vi "RT Main.vi"() -> ()   [LabVIEW 2014]
uses:
  controls/FPGA VI Reference.ctl
  Globals/Global - All RT Loop Stop.vi
  Globals/Global - Monitoring Variables.vi
  Globals/Global - Configuration Options.vi
  support/Message Queue/Message Queue.lvlib
  <vilib>/nisyscfg/nisyscfg.lvlib
  controls/Master Configuration.ctl
  controls/EPICS Configuration.ctl
panel:
  in  "Index":u32
  in  "Message":string
  in  "Send":bool
  in  "stop":bool
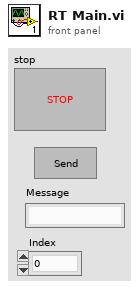
[diagram p1: front panel]
types:
  T1 = typedef "FPGA VI Reference.ctl" = refnum<k20>
  T2 = typedef "Master Configuration.ctl" = cluster{"Epics Configuration":T3, "Epics Configuration File":string, "Number of Channels":u8, "Data rate":u32, "PM Buffer Size":u32}
  T3 = typedef "EPICS Configuration.ctl" = cluster{"DIN Mask":bool[], "# Samples Post Trig":u32, "Armed":bool, "ADC Mask":bool[], "ADC Max Threshold":dbl[], "ADC Min Threshold":dbl[]}
  T4 = typedef "Message Queue.lvlib/All Real-Time Message Queues.ctl" = cluster{"Message Handler":refnum<queue>, "FPGA Subsystem":refnum<queue>}
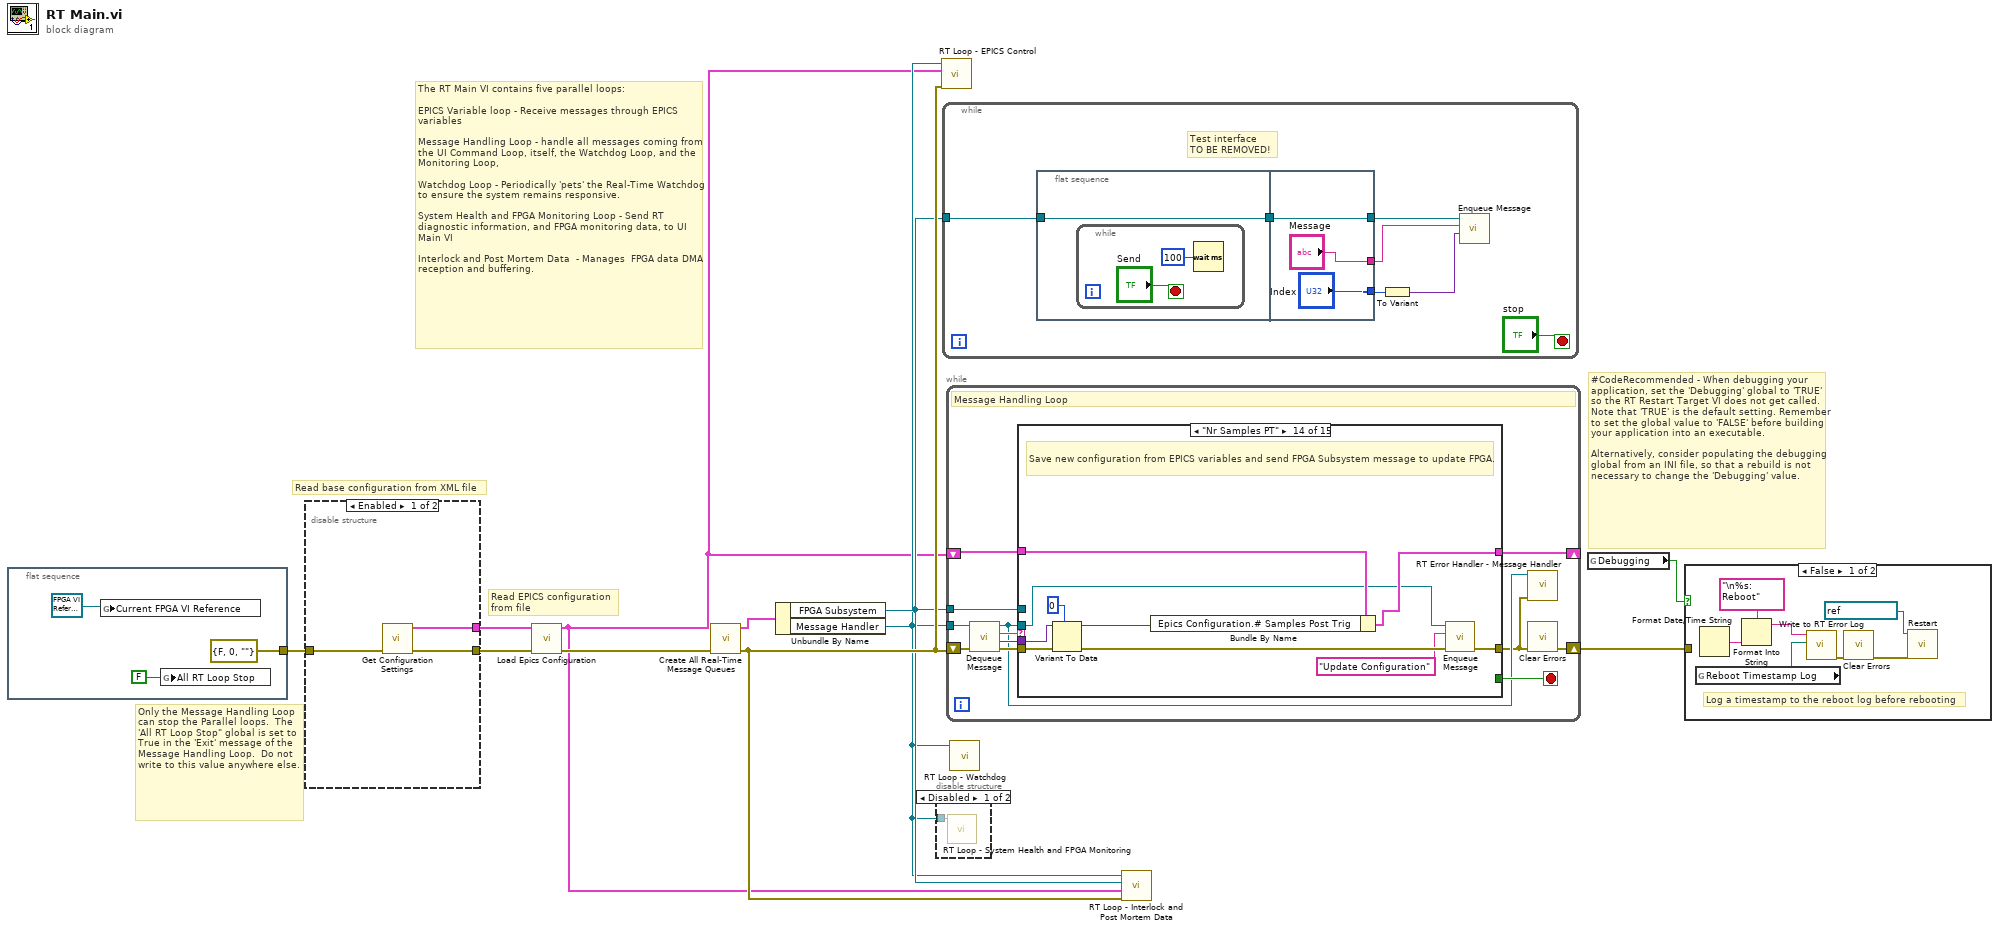
[diagram p0: block diagram]
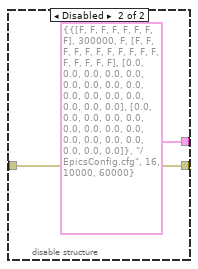
[diagram p3: hidden frame]
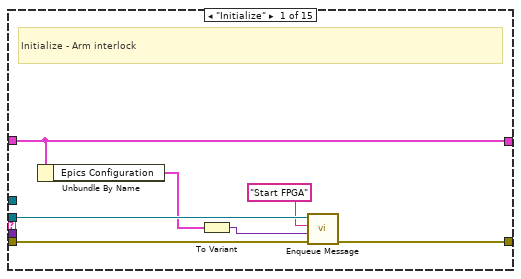
[diagram p5: hidden frame]
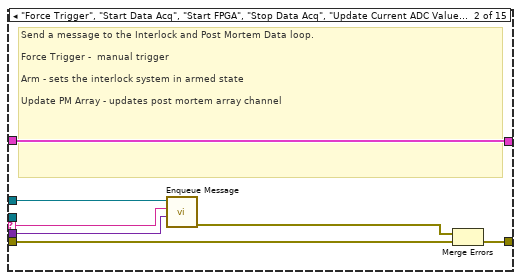
[diagram p6: hidden frame]
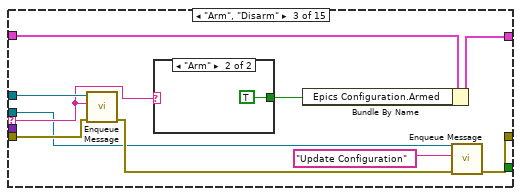
[diagram p7: hidden frame]
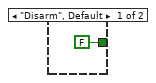
[diagram p8: hidden frame]
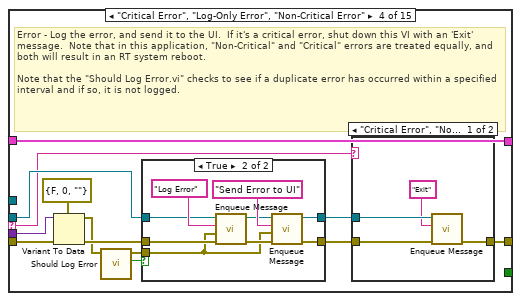
[diagram p9: hidden frame]
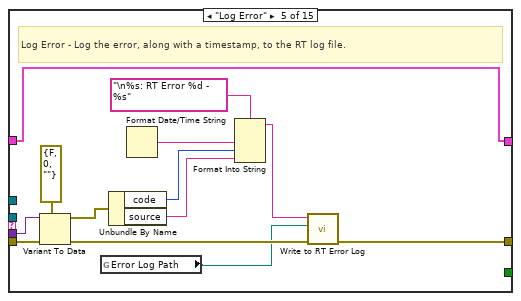
[diagram p12: hidden frame]
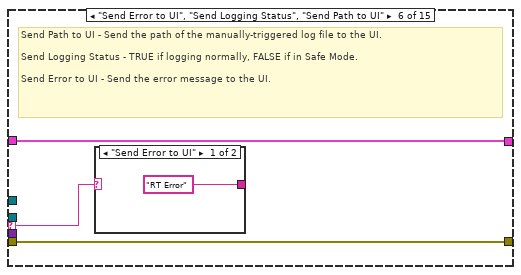
[diagram p13: hidden frame]
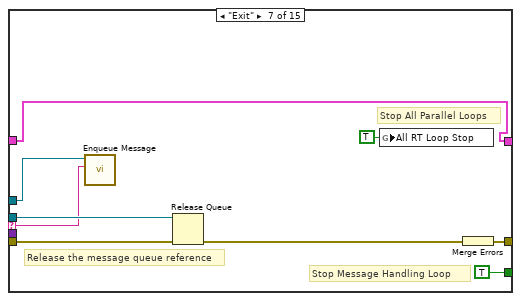
[diagram p15: hidden frame]
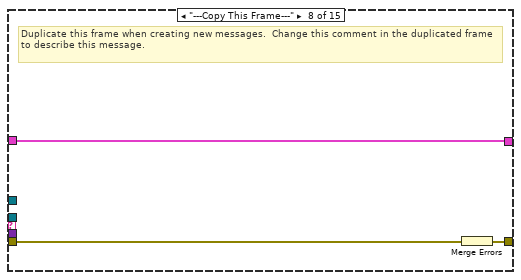
[diagram p16: hidden frame]
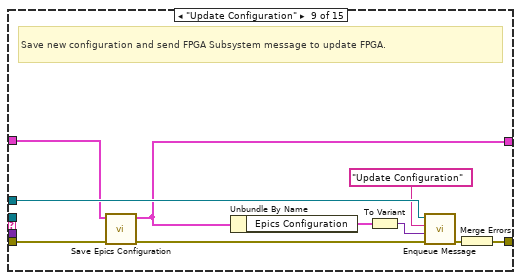
[diagram p17: hidden frame]
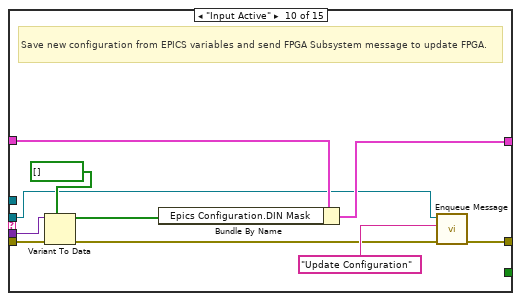
[diagram p18: hidden frame]
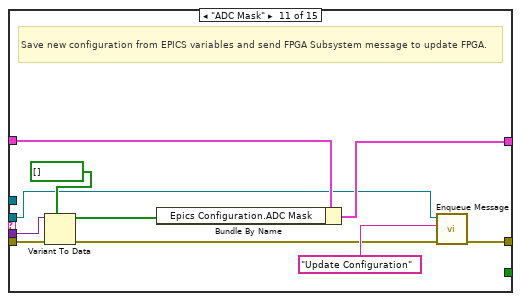
[diagram p19: hidden frame]
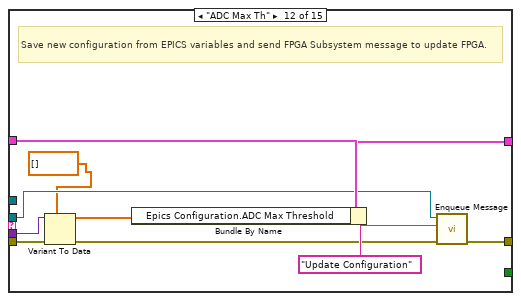
[diagram p20: hidden frame]
diagram:
  # "Read EPICS configuration\nfrom file"
  # "Read base configuration from XML file"
  # "#CodeRecommended - When debugging your application, set the 'Debugging' global to 'TRUE' so the RT Restart Target VI does not get called.  Note that 'TRUE' is the default setting. Remember to set the global value to 'FALSE' before building your application into an executable.\n\nAlternatively, consider populating the debugging global from an INI file, so that a rebuild is not necessary to change the 'Debugging' value."
  # "The RT Main VI contains five parallel loops:\n\nEPICS Variable loop - Receive messages through EPICS variables\n\nMessage Handling Loop - handle all messages coming from the UI Command Loop, itself, the Watchdog Loop, and the Monitoring Loop, \n\nWatchdog Loop - Periodically 'pets' the Real-Time Watchdog to ensure the system remains responsive.\n\nSystem Health and FPGA Monitoring Loop - Send RT diagnostic information, and FPGA monitoring data, to UI Main VI\n\nInterlock and Post Mortem Data  - Manages  FPGA data DMA reception and buffering."
  # "Only the Message Handling Loop can stop the Parallel loops.  The 'All RT Loop Stop\" global is set to True in the 'Exit' message of the Message Handling Loop.  Do not write to this value anywhere else."
  n1 = flat-sequence {
    tunnel: [errorcluster {"status"=FALSE, "code"=0, "source"=""} ("error constant")] -> w11
    frame #0 {
      n2 = global write "Global - Monitoring Variables.vi" "Current FPGA VI Reference"(T1 refnum ("Current FPGA VI Reference")) -> ()
      n3 = global write "Global - All RT Loop Stop.vi" "All RT Loop Stop"(FALSE) -> ()
    }
  }
  n4 = disable-structure shown="Enabled" {
    disable-tunnel: w11 -> [w17 w18]
    disable-tunnel: [w16 w18] -> w5
    disable-tunnel: [w15 T2 {"Epics Configuration"={"DIN Mask"=[FALSE, FALSE, FALSE, FALSE, FALSE, FALSE, FALSE, FALSE], "# Samples Post Trig"=300000, "Armed"=FALSE, "ADC Mask"=[FALSE, FALSE, FALSE, FALSE, FALSE, FALSE, FALSE, FALSE, FALSE, FALSE, FALSE, FALSE, FALSE, FALSE, FALSE, FALSE], "ADC Max Threshold"=[0.0, 0.0, 0.0, 0.0, 0.0, 0.0, 0.0, 0.0, 0.0, 0.0, 0.0, 0.0, 0.0, 0.0, 0.0, 0.0], "ADC Min Threshold"=[0.0, 0.0, 0.0, 0.0, 0.0, 0.0, 0.0, 0.0, 0.0, 0.0, 0.0, 0.0, 0.0, 0.0, 0.0, 0.0]}, "Epics Configuration File"="/EpicsConfig.cfg", "Number of Channels"=16, "Data rate"=10000, "PM Buffer Size"=60000} ("Acquisition and Logging Configuration")] -> w3
    frame Enabled {
      n5 = call "Get Configuration Settings.vi"("error in (no error)"=w17) -> ("error out"=w16:errorcluster, "Acquisition and Logging Configuration"=w15:T2)  [unwired: 9 in]
    }
    frame Disabled {
    }
  }
  n6 = call "Load Epics Configuration.vi"("error in (no error)"=w5, "Master Configuration in"=w3) -> ("error out"=w4:errorcluster, "Master Configuration out"=w1:T2)  [unwired: 8 in]
  n7 = call "Create All Real-Time Message Queues.vi"("error in (no error)"=w4) -> ("error out"=w7:errorcluster, "Message Queues out"=w8:T4)  [unwired: 9 in]
  n8 = Unbundle By Name(w8) -> ("FPGA Subsystem"=w6:refnum<queue>, "Message Handler"=w2:refnum<queue>)
  n9 = disable-structure shown="Disabled" {
    disable-tunnel: w2 -> [w20 _]
    frame Disabled {
      n10 = call "RT Loop - System Health and FPGA Monitoring.vi"("Message Queue"=w20) -> ()  [unwired: 11 in]
    }
    frame Enabled {
    }
  }
  n11 = call "RT Loop - EPICS Control.vi"("Error"=w7, "Acquisition and Logging Configuration"=w1, "Message Handler"=w2) -> ()  [unwired: 9 in]
  n12 = while {
    tunnel: w6 -> [w26]
    stop <- "stop" stop-if-true
    # "Test interface\nTO BE REMOVED!"
    n13 = flat-sequence {
      tunnel: w26 -> [w28]
      tunnel: [w28] -> w24
      tunnel: [w33] -> w25
      tunnel: w24 -> [w33]
      tunnel: ["Message"] -> w23
      tunnel: ["Index"] -> w22
      frame #0 {
        n14 = while {
          stop <- "Send" stop-if-true
          n15 = Wait (ms)(milliseconds to wait=u32 100) -> ()  [unwired: 1 out]
        }
      }
      frame #1 {
      }
    }
    n16 = To Variant(anything=w22) -> (Variant=w21:variant)
    n17 = call "Enqueue Message.vi"("Message Data"=w21, "Message"=w23, "Message Queue"=w25) -> ()  [unwired: 7 in, 2 out]
  }
  n18 = while {
    tunnel: w2 -> [w40]
    shift-right: [w38] -> w10
    shift-left: w7 -> [w44]
    tunnel: w6 -> [w36]
    shift-right: [w34] -> _
    shift-left: w1 -> [w35]
    stop <- w45 stop-if-true
    # "Message Handling Loop"
    n19 = call "Dequeue Message.vi"("error in (no error)"=w44, "Message Queue"=w40) -> ("error out"=w43:errorcluster, "Message Data"=w41:variant, "Message"=w42:string, "dup Message Queue"=w39:refnum<queue>)  [unwired: 6 in]
    n20 = case "Message Cases" shown="\"Nr Samples PT\"" w42 {
      selector: w42 -> [_ w57 w68 w78 _ w115 w120 _ _ _ _ _ _ _ w194]
      tunnel: w39 -> [w52 _ w64 w79 _ _ w127 _ _ w141 w151 w162 w172 w181 _]
      tunnel: w43 -> [w51 w59 w66 w81 w113 w116 w123 w130 w134 w150 w160 w170 w180 w189 _]
      tunnel: [w50 w56 w63 w84 w104 w116 w124 w129 w140 w143 w153 w164 w174 w186 w192] -> w37
      tunnel: [_ _ _ _ _ _ TRUE _ _ _ _ _ _ _ _] -> w45
      tunnel: w41 -> [_ w53 _ w73 w112 _ _ _ _ w149 w159 w169 w179 w188 _]
      tunnel: w36 -> [_ w58 w69 _ _ _ w121 _ w138 _ _ _ _ _ _]
      tunnel: w35 -> [w48 w54 w60 w72 w101 w114 w119 w128 w135 w148 w158 w168 w178 w187 w190]
      tunnel: [w48 w54 w61 w72 w101 w114 w119 w128 w133 w142 w152 w163 w173 w182 w190] -> w34
      frame "Initialize" {
        # "Initialize - Arm interlock"
        n21 = Unbundle By Name(w48) -> ("Epics Configuration"=w47:T3)
        n22 = To Variant(anything=w47) -> (Variant=w46:variant)
        n23 = call "Enqueue Message.vi"("error in (no error)"=w51, "Message Data"=w46, "Message"="Start FPGA", "Message Queue"=w52) -> ("error out"=w50:errorcluster)  [unwired: 6 in, 1 out]
      }
      frame "Force Trigger", "Start Data Acq", "Start FPGA", "Stop Data Acq", "Update Current ADC Values", "Update PM Array" {
        # "Send a message to the Interlock and Post Mortem Data loop.\n\nForce Trigger -  manual trigger\n\nArm - sets the interlock system in armed state\n\nUpdate PM Array - updates post mortem array channel"
        n24 = call "Enqueue Message.vi"("Message Data"=w53, "Message"=w57, "Message Queue"=w58) -> ("error out"=w55:errorcluster)  [unwired: 7 in, 1 out]
        n25 = Merge Errors(w55, w59) -> (w56:errorcluster)
      }
      frame "Arm", "Disarm" {
        n26 = call "Enqueue Message.vi"("error in (no error)"=w66, "Message"=w68, "Message Queue"=w69) -> ("error out"=w65:errorcluster)  [unwired: 7 in, 1 out]
        n27 = case shown="\"Arm\"" w68 {
          tunnel: [FALSE ("Armed") TRUE ("Armed")] -> w67
          frame "Disarm", Default {
          }
          frame "Arm" {
          }
        }
        n28 = Bundle By Name(cluster=w60, "Epics Configuration.Armed"=w67) -> (w61:T2)
        n29 = call "Enqueue Message.vi"("error in (no error)"=w65, "Message"="Update Configuration", "Message Queue"=w64) -> ("error out"=w63:errorcluster)  [unwired: 7 in, 1 out]
      }
      frame "Critical Error", "Log-Only Error", "Non-Critical Error" {
        # "Error - Log the error, and send it to the UI.  If it's a critical error, shut down this VI with an 'Exit' message.  Note that in this application, \"Non-Critical\" and \"Critical\" errors are treated equally, and both will result in an RT system reboot.\n\nNote that the \"Should Log Error.vi\" checks to see if a duplicate error has occurred within a specified interval and if so, it is not logged."
        n30 = Variant To Data(error in=w81, type=errorcluster {"status"=FALSE, "code"=0, "source"=""} ("error out"), Variant=w73) -> (data=w76:errorcluster, error out=w82:errorcluster)
        n31 = call "Should Log Error.vi"("error to report"=w76) -> ("Should Log Error?"=w74:bool, "dup error to report"=w75:errorcluster)  [unwired: 9 in]
        n32 = case shown="True" w74 {
          tunnel: [w86 w93] -> w80
          tunnel: [w85 w92] -> w77
          tunnel: w79 -> [w85 w91]
          tunnel: w82 -> [w86 w88]
          tunnel: w75 -> [_ w87]
          frame False {
          }
          frame True {
            n33 = call "Enqueue Message.vi"("error in (no error)"=w88, "Message Data"=w87, "Message"="Log Error", "Message Queue"=w91) -> ("error out"=w89:errorcluster, "dup Message Queue"=w90:refnum<queue>)  [unwired: 6 in]
            n34 = call "Enqueue Message.vi"("error in (no error)"=w89, "Message Data"=w87, "Message"="Send Error to UI", "Message Queue"=w90) -> ("error out"=w93:errorcluster, "dup Message Queue"=w92:refnum<queue>)  [unwired: 6 in]
          }
        }
        n35 = case shown="\"Critical Error\", \"Non-Critical Error\"" w78 {
          tunnel: w80 -> [w99 w100]
          tunnel: w77 -> [w97 _]
          tunnel: [w98 w100] -> w84
          frame "Critical Error", "Non-Critical Error" {
            n36 = call "Enqueue Message.vi"("error in (no error)"=w99, "Message"="Exit", "Message Queue"=w97) -> ("error out"=w98:errorcluster)  [unwired: 7 in, 1 out]
          }
          frame Default {
          }
        }
      }
      frame "Log Error" {
        # "Log Error - Log the error, along with a timestamp, to the RT log file."
        n37 = Variant To Data(error in=w113, type=errorcluster {"status"=FALSE, "code"=0, "source"=""} ("error constant"), Variant=w112) -> (data=w107:errorcluster, error out=w110:errorcluster)
        n38 = global read "Global - Configuration Options.vi" "Error Log Path"() -> (w102:path)
        n39 = Unbundle By Name(w107) -> ("code"=w106:i32, "source"=w105:string)
        n40 = Format Date/Time String() -> (date/time string=w108:string)  [unwired: 3 in]
        n41 = Format Into String(format string="\n%s: RT Error %d - %s", w108, w106, w105) -> (resulting string=w103:string)  [unwired: 2 in, 1 out]
        n42 = call "Write to RT Error Log.vi"("error in (no error)"=w110, "Error Log Path"=w102, "Log Entry"=w103) -> ("error out"=w104:errorcluster)  [unwired: 8 in]
      }
      frame "Send Error to UI", "Send Logging Status", "Send Path to UI" {
        # "Send Path to UI - Send the path of the manually-triggered log file to the UI.\n\nSend Logging Status - TRUE if logging normally, FALSE if in Safe Mode.\n\nSend Error to UI - Send the error message to the UI."
        n43 = case shown="\"Send Error to UI\"" w115 {
          selector: w115 -> [_ w118]
          tunnel: ["RT Error" ("Message") w118] -> _
          frame "Send Error to UI" {
          }
          frame Default {
          }
        }
      }
      frame "Exit" {
        # "Stop Message Handling Loop"
        # "Stop All Parallel Loops"
        # "Release the message queue reference"
        n44 = call "Enqueue Message.vi"("Message"=w120, "Message Queue"=w121) -> ()  [unwired: 8 in, 2 out]
        n45 = Release Queue(queue=w127, error in (no error)=w123) -> (error out=w125:errorcluster)  [unwired: 1 in, 2 out]
        n46 = global write "Global - All RT Loop Stop.vi" "All RT Loop Stop"(TRUE ("Stop Monitoring Loops")) -> ()
        n47 = Merge Errors(w125) -> (w124:errorcluster)
      }
      frame "---Copy This Frame---" {
        # "Duplicate this frame when creating new messages.  Change this comment in the duplicated frame to describe this message."
        n48 = Merge Errors(w130) -> (w129:errorcluster)
      }
      frame "Update Configuration" {
        # "Save new configuration and send FPGA Subsystem message to update FPGA."
        n49 = call "Save Epics Configuration.vi"("error in (no error)"=w134, "Master Configuration in"=w135) -> ("error out"=w136:errorcluster, "Master Configuration out"=w133:T2)  [unwired: 8 in]
        n50 = Unbundle By Name(w133) -> ("Epics Configuration"=w131:T3)
        n51 = To Variant(anything=w131) -> (Variant=w132:variant)
        n52 = call "Enqueue Message.vi"("error in (no error)"=w136, "Message Data"=w132, "Message"="Update Configuration", "Message Queue"=w138) -> ("error out"=w139:errorcluster)  [unwired: 6 in, 1 out]
        n53 = Merge Errors(w139) -> (w140:errorcluster)
      }
      frame "Input Active" {
        # "Save new configuration from EPICS variables and send FPGA Subsystem message to update FPGA."
        n54 = Variant To Data(error in=w150, type=bool[] [] ("Epics Configuration.Input active"), Variant=w149) -> (data=w146:bool[], error out=w144:errorcluster)
        n55 = Bundle By Name(cluster=w148, "Epics Configuration.DIN Mask"=w146) -> (w142:T2)
        n56 = call "Enqueue Message.vi"("error in (no error)"=w144, "Message"="Update Configuration", "Message Queue"=w141) -> ("error out"=w143:errorcluster)  [unwired: 7 in, 1 out]
      }
      frame "ADC Mask" {
        # "Save new configuration from EPICS variables and send FPGA Subsystem message to update FPGA."
        n57 = Variant To Data(error in=w160, type=bool[] [] ("Epics Configuration.Input active"), Variant=w159) -> (data=w156:bool[], error out=w154:errorcluster)
        n58 = Bundle By Name(cluster=w158, "Epics Configuration.ADC Mask"=w156) -> (w152:T2)
        n59 = call "Enqueue Message.vi"("error in (no error)"=w154, "Message"="Update Configuration", "Message Queue"=w151) -> ("error out"=w153:errorcluster)  [unwired: 7 in, 1 out]
      }
      frame "ADC Max Th" {
        # "Save new configuration from EPICS variables and send FPGA Subsystem message to update FPGA."
        n60 = Variant To Data(error in=w170, type=dbl[] [] ("Epics Configuration.ADC Max Threshold"), Variant=w169) -> (data=w167:dbl[], error out=w165:errorcluster)
        n61 = Bundle By Name(cluster=w168, "Epics Configuration.ADC Max Threshold"=w167) -> (w163:T2)
        n62 = call "Enqueue Message.vi"("error in (no error)"=w165, "Message"="Update Configuration", "Message Queue"=w162) -> ("error out"=w164:errorcluster)  [unwired: 7 in, 1 out]
      }
      frame "ADC Min Th" {
        # "Save new configuration from EPICS variables and send FPGA Subsystem message to update FPGA."
        n63 = Variant To Data(error in=w180, type=dbl[] [] ("Epics Configuration.ADC Max Threshold"), Variant=w179) -> (data=w177:dbl[], error out=w175:errorcluster)
        n64 = Bundle By Name(cluster=w178, "Epics Configuration.ADC Min Threshold"=w177) -> (w173:T2)
        n65 = call "Enqueue Message.vi"("error in (no error)"=w175, "Message"="Update Configuration", "Message Queue"=w172) -> ("error out"=w174:errorcluster)  [unwired: 7 in, 1 out]
      }
      frame "Nr Samples PT" {
        # "Save new configuration from EPICS variables and send FPGA Subsystem message to update FPGA."
        n66 = Variant To Data(error in=w189, type=u32 0 ("Epics Configuration.# Samples Post Trig"), Variant=w188) -> (data=w184:u32, error out=w186:errorcluster)
        n67 = Bundle By Name(cluster=w187, "Epics Configuration.# Samples Post Trig"=w184) -> (w182:T2)
        n68 = call "Enqueue Message.vi"("Message"="Update Configuration", "Message Queue"=w181) -> ()  [unwired: 8 in, 2 out]
      }
      frame Default {
        # "'Default' case only runs if there is a message that isn't defined in any of the other cases.  Output a programming error."
        n69 = Format Into String(format string="The invalid message string \"%s\" was received in the Message Handling Loop." ("Unknown Message Error Text"), w194) -> (resulting string=w191:string)  [unwired: 2 in, 1 out]
        n70 = call <vilib>:"Error Cluster From Error Code.vi"("error message (\"\")"=w191, "error code (0)"=1) -> ("error out"=w192:errorcluster)  [unwired: 7 in]
      }
    }
    n71 = call "RT Error Handler - Message Handler.vi"("error in (no error)"=w37, "Message Queue"=w39) -> ()  [unwired: 9 in, 1 out]
    n72 = call <vilib>:"Clear Errors.vi"("error in (no error)"=w37) -> ("error out"=w38:errorcluster)  [unwired: 5 in, 1 out]
  }
  n73 = call "RT Loop - Watchdog.vi"("Message Queue"=w2) -> ()  [unwired: 11 in]
  n74 = call "RT Loop - Interlock and Post Mortem Data.vi"("error in (no error)"=w7, "Master Configuration"=w1, "FPGA Subsystem"=w6, "Message Handler"=w2) -> ()  [unwired: 8 in]
  n75 = global read "Global - Configuration Options.vi" "Debugging"() -> (w9:bool)
  n76 = case shown="False" w9 {
    tunnel: w10 -> [_ _]
    frame False {
      # "Log a timestamp to the reboot log before rebooting"
      n77 = global read "Global - Configuration Options.vi" "Reboot Timestamp Log"() -> (w198:path)
      n78 = Format Date/Time String() -> (date/time string=w200:string)  [unwired: 3 in]
      n79 = Format Into String(format string="\n%s: Reboot", w200) -> (resulting string=w199:string)  [unwired: 2 in, 1 out]
      n80 = call "Write to RT Error Log.vi"("Error Log Path"=w198, "Log Entry"=w199) -> ("error out"=w202:errorcluster)  [unwired: 9 in]
      n81 = call <vilib>:"Clear Errors.vi"("error in (no error)"=w202) -> ("error out"=w197:errorcluster)  [unwired: 5 in, 1 out]
      n82 = call <vilib>:"Restart.vi"("error in (no error)"=w197, "Session in"=refnum<k21> "localhost" ("session in")) -> ()  [unwired: 7 in, 3 out]
    }
    frame True {
    }
  }
